vi "ActivateSole.vi"(9 "String":string, 10 "Extend":bool, 11 "Retract":bool) -> ()   [LabVIEW 2015]
uses:
  <vilib>/Rock Robotics/WPI/Solenoid/WPI_SolenoidValue.ctl
  <vilib>/Rock Robotics/Network Tables/NT Write Boolean.vi
  <vilib>/Rock Robotics/WPI/Solenoid/WPI_SolenoidSetEnum.vi
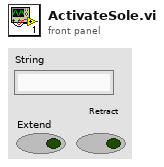
[diagram p1: front panel]
types:
  T1 = typedef "WPI_SolenoidValue.ctl" = enum16{"Off", "On", "Forward", "Reverse"}
  T2 = typedef "WPI_SolenoidDevRef.ctl" = cluster{"DevStatus":errorcluster, "Pneumatics Control Module":u8, "Forward Solenoid Channel":T3, "Reverse Solenoid Channel":T3}
  T3 = typedef "WPI_SolenoidChannel.ctl" = enum8{"Solenoid 0", "Solenoid 1", "Solenoid 2", "Solenoid 3", "Solenoid 4", "Solenoid 5", "Solenoid 6", "Solenoid 7", "Invalid"}
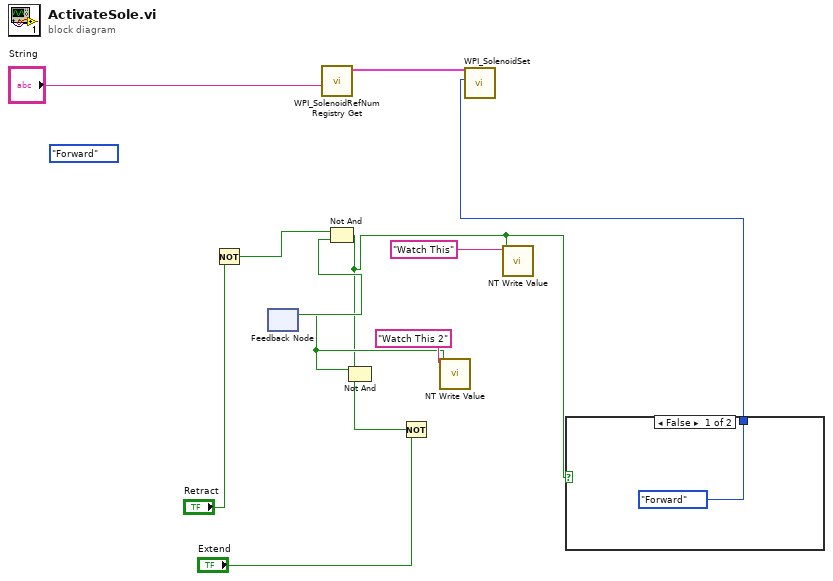
[diagram p0: block diagram]
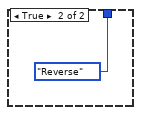
[diagram p2: hidden frame]
diagram:
  (unwired) WPI_SolenoidValue."Forward" ("Value")
  n1 = Not(x="Retract") -> (.not. x?=w8:bool)
  n2 = feedback #1() -> (w10:bool)  [unwired: 1 in]
  n3 = call <vilib>:"WPI_SolenoidRefNum Registry Get.vi"("refnum name"="String") -> ("SolenoidDevRef"=w12:T2)  [unwired: 9 in, 1 out]
  n4 = Not And(1:w10, 2:w8) -> (0:w2:bool)
  n5 = Not(x="Extend") -> (.not. x?=w5:bool)
  n6 = Not And(1:w5, 2:w2) -> (0:w6:bool)
  n7 = feedback-in #1(w6) -> ()
  n8 = call-poly <vilib>:"NT Write Value.vi"("Boolean"=w6, "Name"="Watch This 2") -> ()  [unwired: 9 in, 1 out]
  n9 = call-poly <vilib>:"NT Write Value.vi"("Boolean"=w2, "Name"="Watch This") -> ()  [unwired: 9 in, 1 out]
  n10 = case shown="False" w2 {
    tunnel: [WPI_SolenoidValue."Forward" ("Value") WPI_SolenoidValue."Reverse" ("Value")] -> w3
    frame False {
    }
    frame True {
    }
  }
  n11 = call-poly <vilib>:"WPI_SolenoidSet.vi"("Value"=w3, "SolenoidDevRef"=w12) -> ()  [unwired: 1 in, 9 out]
